vi "niRFUtil FTW Generate VBW IIR Filter.vi"(1 "Sampling Period (sec)":dbl format="%^.2e", 2 "VBW (Hz)":dbl format="%^.2e") -> (0 "VBW Filter":T1 {"Group Delay (sec)" format="%^.2e"; "Filter"."Forward Coefficients" format="%.4f"; "Filter"."Reverse Coefficients" format="%.4f"})   [LabVIEW 2015, in "niRFUtil.lvlib"]
doc: "(c) Copyright 2006, National Instruments, Inc. This VI may not be duplicated, sold, or distributed without written consent from National Instruments."
uses:
  niRFUtil.lvlib
  Includes/niRFUtil INC IIR Filter.ctl
  <vilib>/Analysis/NI_AALBase.lvlib
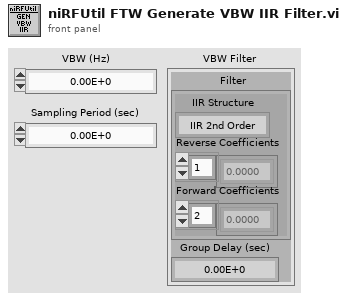
[diagram p1: front panel]
types:
  T1 = typedef "niRFUtil.lvlib/niRFUtil INC IIR Filter.ctl" = cluster{"Filter":cluster{"IIR Structure":enum32{"IIR 2nd Order", "IIR 4th Order"}, "Reverse Coefficients":dbl[], "Forward Coefficients":dbl[]}, "Group Delay (sec)":dbl}
  T2 = enum32{"Lowpass", "Highpass", "Bandpass", "Bandstop"}
  T3 = cluster{"Sampling Period (sec)":dbl, "VBW (Hz)":dbl}
  T4 = cluster{"filter structure":enum32{"IIR 2nd Order", "IIR 4th Order"}, "Reverse Coefficients":dbl[], "Forward Coefficients":dbl[]}
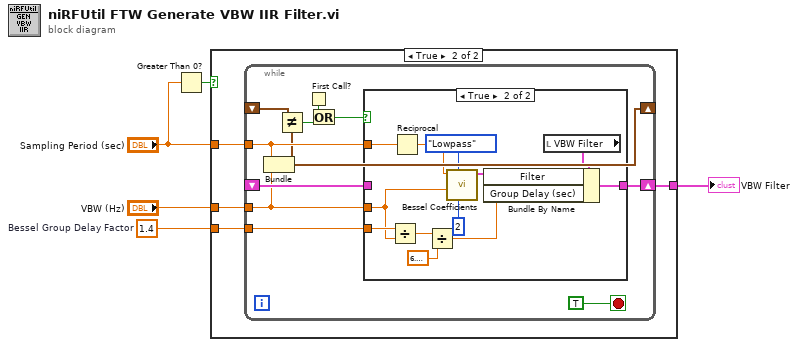
[diagram p0: block diagram]
diagram:
  w4 = 1.4  # Bessel Group Delay Factor
  n1 = Greater Than 0?(x="Sampling Period (sec)") -> (x > 0?=w1:bool)
  n2 = case shown="True" w1 {
    tunnel: "Sampling Period (sec)" -> [_ w9]
    tunnel: [_ w8] -> w5
    tunnel: w4 -> [_ w7]
    tunnel: "VBW (Hz)" -> [_ w6]
    frame False {
    }
    frame True {
      n3 = while {
        tunnel: w9 -> [w14]
        tunnel: w7 -> [w19]
        tunnel: w6 -> [w13]
        shift-right: [w20] -> w8
        shift-left: _ -> [w17]
        shift-right: [w11] -> _
        shift-left: _ -> [w12]
        stop <- TRUE stop-if-true
        n4 = Bundle("Sampling Period (sec)"=w14, "VBW (Hz)"=w13) -> (w11:T3)  [unwired: 1 out]
        n5 = Not Equal?(x=w12, y=w11) -> (x != y?=w16:bool)
        n6 = First Call?() -> (First Call?: T/F=w15:bool)
        n7 = Or(x=w15, y=w16) -> (x .or. y?=w10:bool)
        n8 = case shown="True" w10 {
          tunnel: w14 -> [_ w33]
          tunnel: [w21 w32] -> w20
          tunnel: w19 -> [_ w31]
          tunnel: w13 -> [_ w30]
          tunnel: w17 -> [w21 _]
          frame False {
          }
          frame True {
            n9 = Divide(x=w31, y=w30) -> (x/y=w24:dbl)
            n10 = Reciprocal(x=w33) -> (1/x=w25:dbl)
            n11 = Divide(x=w24, y=6.283185307179586) -> (x/y=w22:dbl)
            n12 = call <vilib>:"Bessel Coefficients.vi"("order"=2, "filter type"=T2."Lowpass", "low cutoff freq: fl"=w30, "sampling freq: fs"=w25) -> ("IIR Filter Cluster"=w26:T4)  [unwired: 6 in, 1 out]
            n13 = local read "VBW Filter"() -> (w27:T1)
            n14 = Bundle By Name(cluster=w27, "Filter"=w26, "Group Delay (sec)"=w22) -> (w32:T1)
          }
        }
      }
    }
  }
  "VBW Filter" <- w5
